vi "rotate.vi"(3 "Roll":dbl, 4 "Yaw":dbl, 5 "Pitch":dbl) -> (0 "NewRoll":dbl, 1 "NewYaw":dbl, 2 "NewPitch":dbl)   [LabVIEW 2012]
uses:
  <vilib>/imath/engines/lvmath2/RunTimeEngine/ErrorHandling/NIMS_Finalize Error.vi
  <vilib>/imath/engines/lvmath2/RunTimeEngine/NodeEndStatement/NIMS_NodeEndStatement_Output.vi
  <instcachedir>/0/NIMS_NodeEndStatement_Output_53EC0D466D134D7ABD903AC30B43404B.lvgen/NIMS_NodeEndStatement_Output_53EC0D466D134D7ABD903AC30B43404B_001.vi
  <vilib>/imath/engines/lvmath2/RunTimeEngine/ArithmeticOperatorToken/NIMS_ArithmeticOperator_multmx(M,CV)-internal.vi
  <instcachedir>/0/NIMS_ArithmeticOperator_multmx(M,CV)-internal_C5AED7E73A244A079B85E565111B9931.lvgen/NIMS_ArithmeticOperator_multmx(M,CV)-internal_C5AED7E73A244A079B85E565111B9931_001.vi
  <vilib>/imathl/engines/lvmath/Functions/Error Handling/Create Error.vi
  <vilib>/imath/engines/lvmath2/RunTimeEngine/VariableToken/Read/NIMS_Get Elements - CV(_) - Check.vi
  <instcachedir>/0/NIMS_Get Elements - CV(_) - Check_9400805D97754C2091B853F6E24C0606.lvgen/NIMS_Get Elements - CV(_) - Check_9400805D97754C2091B853F6E24C0606_001.vi
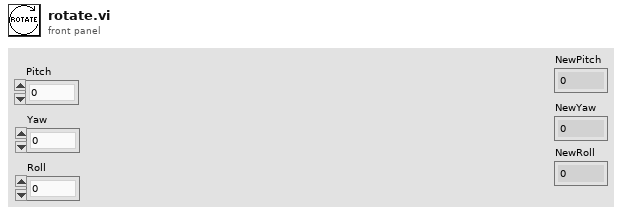
[diagram p1: front panel]
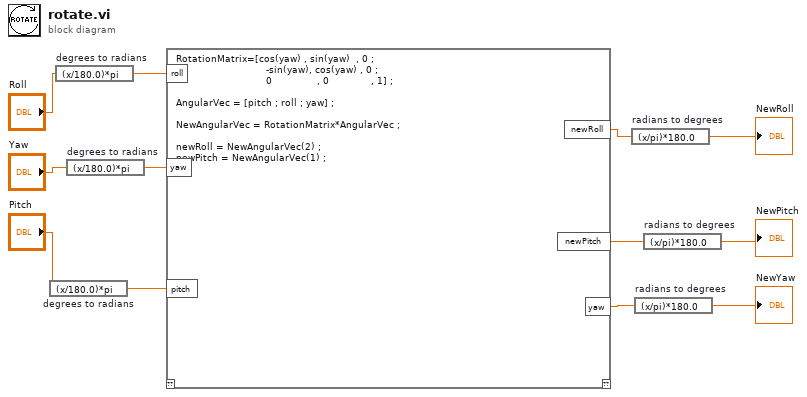
[diagram p0: block diagram]
diagram:
  n1 = expression code="(x/180.0)*pi" "degrees to radians"("Pitch") -> (w4:dbl)
  n2 = expression code="(x/180.0)*pi" "degrees to radians"("Roll") -> (w6:dbl)
  n3 = expression code="(x/180.0)*pi" "degrees to radians"("Yaw") -> (w5:dbl)
  n4 = mathscript code="RotationMatrix=[cos(yaw) , sin(yaw)  , 0 ;\n                              -sin(yaw), cos(yaw) , 0 ;\n                              0               , 0              , 1] ; \n\nAngularVec = [pitch ; roll ; yaw] ;\n\nNewAngularVec = RotationMatrix*AngularVec ;\n\nnewRoll = NewAngularVec(2) ;\nnewPitch = NewAngularVec(1) ;"("roll"=w6, "yaw"=w5, "pitch"=w4) -> ("newRoll"=w9:dbl, "newPitch"=w8:dbl, "yaw"=w7:dbl)  [unwired: 1 in, 1 out]
  n5 = expression code="(x/pi)*180.0" "radians to degrees"(w9) -> (→"NewRoll":dbl)
  n6 = expression code="(x/pi)*180.0" "radians to degrees"(w7) -> (→"NewYaw":dbl)
  n7 = expression code="(x/pi)*180.0" "radians to degrees"(w8) -> (→"NewPitch":dbl)
